vi "_15_Sample_qsns_05[1].vi"() -> ()   [LabVIEW 2020]
panel:
  out "Array":dbl[](array[numeric])
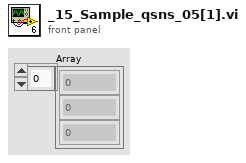
[diagram p1: front panel]
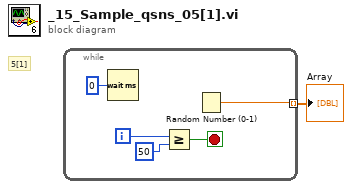
[diagram p0: block diagram]
diagram:
  # "5[1]"
  n1 = while {
    tunnel: [w2] -> w1 mode=indexing
    i -> [w4]
    stop <- w5 stop-if-true
    n2 = Wait (ms)(milliseconds to wait=u32 0) -> ()  [unwired: 1 out]
    n3 = Greater Or Equal?(x=w4, y=50) -> (x >= y?=w5:bool)
    n4 = Random Number (0-1)() -> (number: 0 to 1=w2:dbl)
  }
  "Array" <- w1
